vi "firstVI.vi"() -> ()   [LabVIEW 2017]
panel:
  in  "Knob2":dbl(knob) max=101.0 step=1.0 scale=2.0..100.0 scale format="%#.2f"
  out "Celsius\ngg 2":dbl(slide) scale=0.0..100.0
  in  "This is a switcher":bool
  in  "Fahrenheit":dbl(slide) scale=-25.0..200.0
  out "Celsius\ngg":dbl(slide) scale=0.0..100.0
  # "it seems that this is a comment"
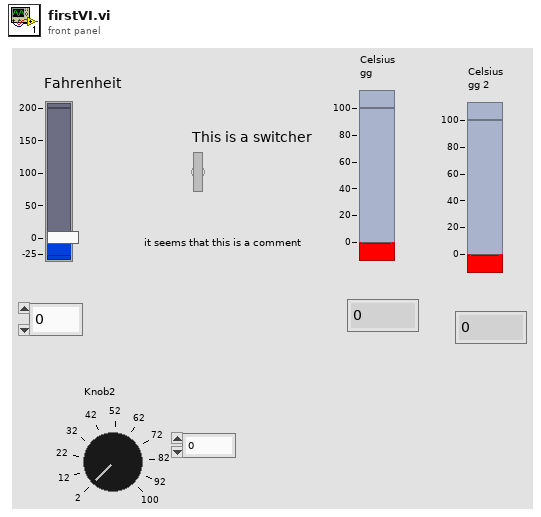
[diagram p1: front panel]
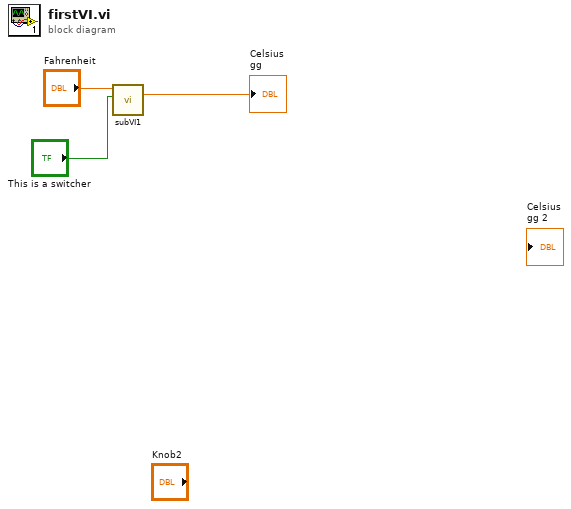
[diagram p0: block diagram]
diagram:
  n1 = call "subVI1.vi"("Boolean"="This is a switcher", "Fahrenheit"="Fahrenheit") -> ("Celsius"=→"Celsius\ngg":dbl)  [unwired: 9 in]
